vi "Get Msg Attributes.vi"(11 "Actor Create Msg Strategy in":refnum<class "Actor Create Msg Strategy.lvclass">) -> (1 "Nest Alias":string, 2 "Nest Actor":refnum<class "Actor.lvclass">)   [LabVIEW 2021, in "Actor Create.lvlib" / "Actor Create Msg Strategy.lvclass"]
uses:
  Actor Create Msg Strategy.lvclass
  LVCAM/Actor/Actor.lvclass
  Actor Create Msg Strategy.lvclass/Actor Create Msg Strategy.ctl
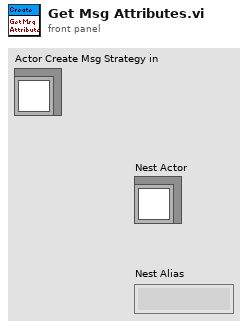
[diagram p1: front panel]
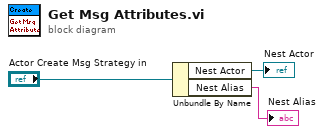
[diagram p0: block diagram]
diagram:
  n1 = Unbundle By Name("Actor Create Msg Strategy in") -> ("Nest Actor"=→"Nest Actor":refnum<class "Actor.lvclass">, "Nest Alias"=→"Nest Alias":string)
